vi "VI AK TCP.vi"(5 "Port changed in":bool, 6 "Aktionen":T1, 8 "error in":errorcluster caption="error out", 10 "Port":u16=3615, 11 "Sprachliste":string[][](array[string])) -> (0 "error out":errorcluster, 3 "connection ID":refnum<k5>)   [LabVIEW 2020, in "AK-Schnittstelle.lvlib" / "AK TCP.lvlib"]
uses:
  AK TCP.lvlib
  Aktionen AK.ctl
  Daten weitergeben Aktionen.ctl
  Aktionen Gespeicherte Werte.ctl
  AK-Schnittstelle.lvlib
  Sprachverwaltung/Sprachverwaltung.lvlib
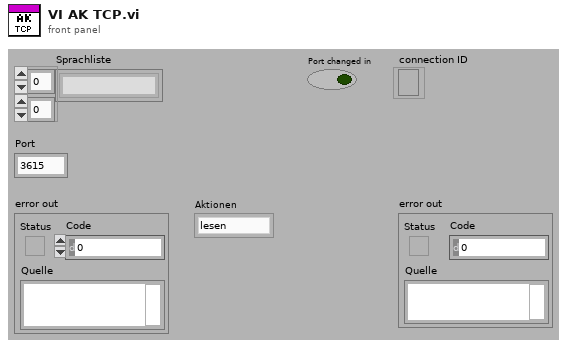
[diagram p1: front panel]
types:
  T1 = typedef "AK-Schnittstelle.lvlib/Aktionen AK.ctl" = enum16{"lesen", "initialisieren", "beenden", "AK Komm"}
  T2 = typedef "AK-Schnittstelle.lvlib/Daten weitergeben Aktionen.ctl" = enum16{"lesen", "schreiben", "Log löschen", "Detail", "Detail löschen", "Speicher Freigeben"}
  T3 = typedef "AK-Schnittstelle.lvlib/Aktionen Gespeicherte Werte.ctl" = enum16{"lesen", "laden", "speichern", "Seriell", "TCP", "Diverse", "AKTIV", "AK-Namen"}
  T4 = typedef "AK-Schnittstelle.lvlib/Diverse gespeicherte Werte.ctl" = cluster{"Kalibriergaseingang":i16, "SamplePoint":i16, "CalGas zu PNS":i16, "Gas-Reihenfolge":i16[], "Zeit 0-Gas":sgl, "Zeit CalGas":sgl, "AK Befehlssatz":T5}
  T5 = typedef "AK-Schnittstelle.lvlib/AK Befehlssatz.ctl" = enum16{"MEXA", "IAG v1.4", "AVL (Puma)", "PEUS"}
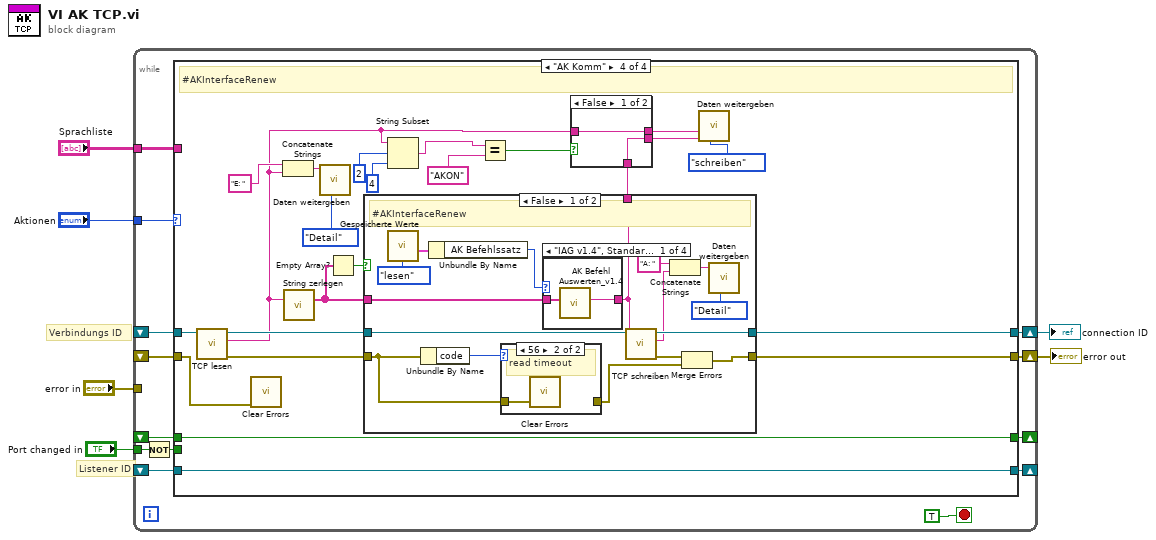
[diagram p0: block diagram]
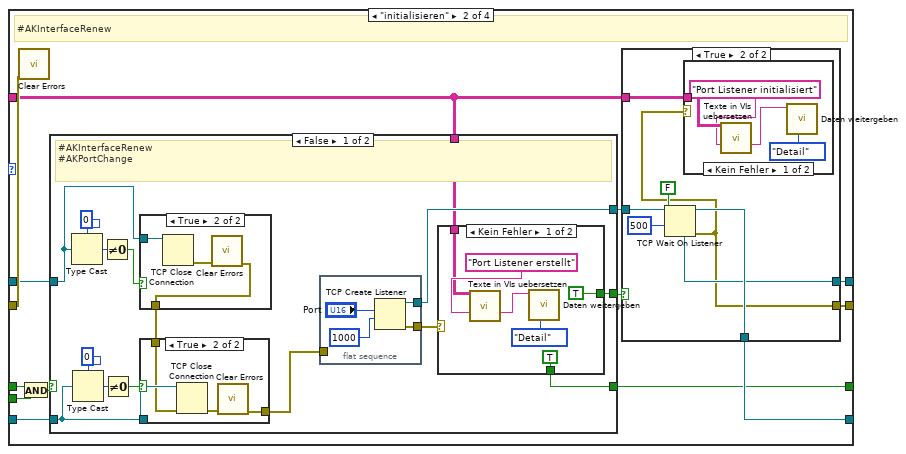
[diagram p3: hidden frame]
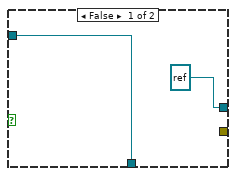
[diagram p4: hidden frame]
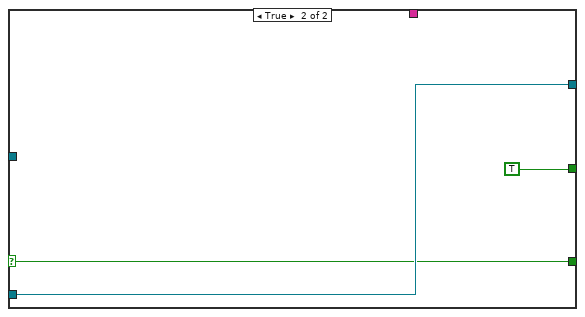
[diagram p9: hidden frame]
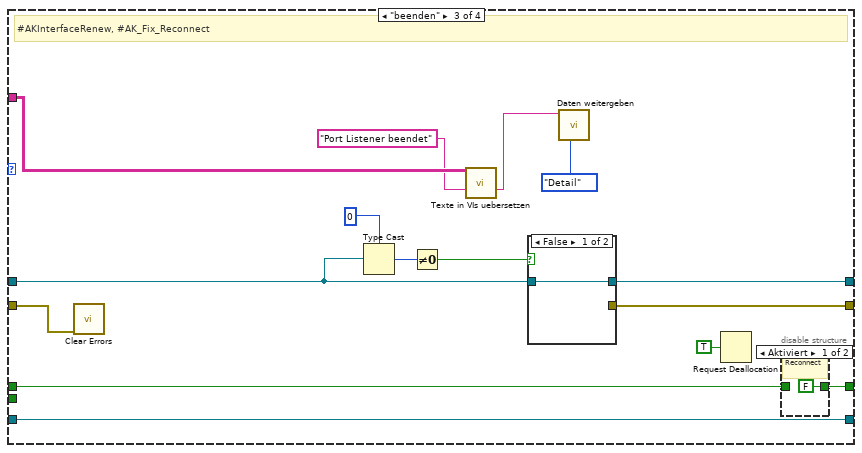
[diagram p10: hidden frame]
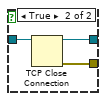
[diagram p11: hidden frame]
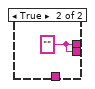
[diagram p13: hidden frame]
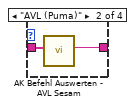
[diagram p15: hidden frame]
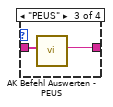
[diagram p16: hidden frame]
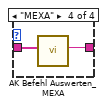
[diagram p17: hidden frame]
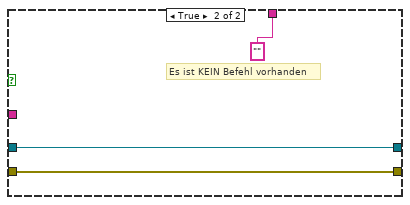
[diagram p18: hidden frame]
diagram:
  # "Verbindungs ID"
  # "Listener ID"
  n1 = while {
    tunnel: "Aktionen" -> [w19]
    shift-right: [w17] -> _
    shift-left: _ -> [w16]
    shift-right: [w18] -> w5
    shift-left: _ -> [w15]
    tunnel: "error in" -> [_]
    shift-right: [w13] -> w3
    shift-left: _ -> [w12]
    shift-right: [w10] -> _
    shift-left: _ -> [w11]
    tunnel: "Port changed in" -> [w9]
    tunnel: "Sprachliste" -> [w7]
    stop <- TRUE stop-if-true
    n2 = Not(x=w9) -> (.not. x?=w8:bool)
    n3 = case shown="\"AK Komm\"" w19 {
      tunnel: [w22 w30 w99 w126] -> w18
      tunnel: [w23 w35 w97 w120] -> w17
      tunnel: w16 -> [w23 w34 w97 w120]
      tunnel: w15 -> [w22 w31 w96 w123]
      tunnel: [w21 w33 w98 w119] -> w13
      tunnel: w12 -> [w21 w26 w89 w121]
      tunnel: w11 -> [w20 w29 w92 w118]
      tunnel: [w20 w32 w93 w118] -> w10
      tunnel: w8 -> [_ w28 _ _]
      tunnel: w7 -> [_ w24 w87 _]
      frame "lesen", Default {
      }
      frame "initialisieren" {
        # "#AKInterfaceRenew"
        n4 = call <vilib>:"Clear Errors.vi"("error in (no error)"=w31) -> ()  [unwired: 5 in, 2 out]
        n5 = And(x=w29, y=w28) -> (x .and. y?=w27:bool)
        n6 = case shown="False" w27 {
          selector: w27 -> [_ w83]
          tunnel: [w64 w84] -> w36
          tunnel: w34 -> [w60 w84]
          tunnel: [w62 w83] -> w32
          tunnel: w26 -> [w54 _]
          tunnel: [w51 TRUE] -> w25
          tunnel: w24 -> [w50 _]
          frame False {
            # "#AKInterfaceRenew\n#AKPortChange"
            n7 = Type Cast(type=u32 0, x=w54) -> (*(type *) &x=w57:u32)
            n8 = Type Cast(type=u32 0, x=w60) -> (*(type *) &x=w61:u32)
            n9 = Not Equal To 0?(x=w57) -> (x != 0?=w55:bool)
            n10 = Not Equal To 0?(x=w61) -> (x != 0?=w59:bool)
            n11 = case shown="True" w55 {
              tunnel: [_ w66] -> w53
              tunnel: w54 -> [_ w65]
              frame False {
              }
              frame True {
                n12 = TCP Close Connection(connection ID=w65) -> (error out=w67:errorcluster)  [unwired: 2 in, 1 out]
                n13 = call <vilib>:"Clear Errors.vi"("error in (no error)"=w67) -> ("error out"=w66:errorcluster)  [unwired: 5 in, 1 out]
              }
            }
            n14 = case shown="True" w59 {
              tunnel: w60 -> [_ w71]
              tunnel: w53 -> [_ w69]
              tunnel: [_ w68] -> w52
              frame False {
              }
              frame True {
                n15 = TCP Close Connection(connection ID=w71, error in (no error)=w69) -> (error out=w70:errorcluster)  [unwired: 1 in, 1 out]
                n16 = call <vilib>:"Clear Errors.vi"("error in (no error)"=w70) -> ("error out"=w68:errorcluster)  [unwired: 5 in, 1 out]
              }
            }
            n17 = flat-sequence {
              tunnel: [w74] -> w64
              tunnel: [w73] -> w63
              tunnel: w52 -> [_]
              frame #0 {
                n18 = TCP Create Listener(9:1000 ("timeout ms (wait forever: -1)"), 10:"Port") -> (0:w73:errorcluster, 3:w74:refnum<k5>)  [unwired: 3 in, 1 out]
              }
            }
            n19 = case shown="Kein Fehler" w63 {
              tunnel: [TRUE _] -> w62
              tunnel: [TRUE _] -> w51
              tunnel: w50 -> [w77 _]
              frame No Error {
                n20 = call "Texte in VIs uebersetzen.vi"("Sprachliste"=w77, "String zum Übersetzen"="Port Listener erstellt" ("Detail")) -> ("String zum Übersetzen"=w76:string)  [unwired: 9 in, 4 out]
                n21 = call "Daten weitergeben.vi"("Aktionen"=Daten_weitergeben_Aktionen."Detail", "Detail"=w76) -> ()  [unwired: 5 in, 5 out]
              }
              frame Error {
              }
            }
          }
          frame True {
          }
        }
        n22 = case shown="True" w25 {
          tunnel: w36 -> [w38 w44]
          tunnel: [w38 w43] -> w35
          tunnel: [refnum<k5> refnum ("listener ID") w42] -> w33
          tunnel: [_ w40] -> w30
          tunnel: w24 -> [_ w39]
          frame False {
          }
          frame True {
            n23 = TCP Wait On Listener(9:500 ("Timeout in ms (kein: -1)"), 10:FALSE ("Auflösen der Netzwerkadresse (T)"), 11:w44) -> (0:w40:errorcluster, 3:w43:refnum<k5>, 4:w42:refnum<k5>)  [unwired: 1 in, 2 out]
            n24 = case shown="Kein Fehler" w40 {
              tunnel: w39 -> [w48 _]
              frame No Error {
                n25 = call "Texte in VIs uebersetzen.vi"("Sprachliste"=w48, "String zum Übersetzen"="Port Listener initialisiert" ("Detail")) -> ("String zum Übersetzen"=w46:string)  [unwired: 9 in, 4 out]
                n26 = call "Daten weitergeben.vi"("Aktionen"=Daten_weitergeben_Aktionen."Detail", "Detail"=w46) -> ()  [unwired: 5 in, 5 out]
              }
              frame Error {
              }
            }
          }
        }
      }
      frame "beenden" {
        # "#AKInterfaceRenew, #AK_Fix_Reconnect"
        n27 = call <vilib>:"Clear Errors.vi"("error in (no error)"=w96) -> ()  [unwired: 5 in, 2 out]
        n28 = Type Cast(type=u32 0, x=w89) -> (*(type *) &x=w91:u32)
        n29 = Not Equal To 0?(x=w91) -> (x != 0?=w88:bool)
        n30 = call "Texte in VIs uebersetzen.vi"("Sprachliste"=w87, "String zum Übersetzen"="Port Listener beendet" ("Detail")) -> ("String zum Übersetzen"=w85:string)  [unwired: 9 in, 4 out]
        n31 = case shown="False" w88 {
          tunnel: [_ w103] -> w99
          tunnel: w89 -> [w100 w102]
          tunnel: [w100 w101] -> w98
          frame False {
          }
          frame True {
            n32 = TCP Close Connection(connection ID=w102) -> (connection ID out=w101:refnum<k5>, error out=w103:errorcluster)  [unwired: 2 in]
          }
        }
        n33 = call "Daten weitergeben.vi"("Aktionen"=Daten_weitergeben_Aktionen."Detail", "Detail"=w85) -> ()  [unwired: 5 in, 5 out]
        n34 = Request Deallocation(TRUE ("Flag")) -> ()
        n35 = disable-structure shown="Aktiviert" {
          disable-tunnel: [FALSE w105] -> w93
          disable-tunnel: w92 -> [_ w105]
          frame Enabled {
            # "#AK_Fix_Reconnect"
          }
          frame Disabled {
          }
        }
      }
      frame "AK Komm" {
        # "#AKInterfaceRenew"
        n36 = call "TCP lesen.vi"("connection ID"=w121) -> ("error out"=w122:errorcluster, "Daten (Ausgang)"=w109:string, "connection ID"=w125:refnum<k5>)  [unwired: 8 in]
        n37 = call <vilib>:"Clear Errors.vi"("error in (no error)"=w123) -> ()  [unwired: 5 in, 2 out]
        n38 = Concatenate Strings("E: ", w109) -> (w116:string)
        n39 = call "String zerlegen.vi"("read buffer"=w109) -> ("Array"=w128:string[])  [unwired: 14 in]
        n40 = call "Daten weitergeben.vi"("Aktionen"=Daten_weitergeben_Aktionen."Detail", "Detail"=w116) -> ()  [unwired: 5 in, 5 out]
        n41 = Empty Array?(array=w128) -> (empty?=w127:bool)
        n42 = case shown="False" w127 {
          tunnel: w128 -> [w145 _]
          tunnel: w125 -> [w147 w160]
          tunnel: [w146 w160] -> w119
          tunnel: [w135 w158] -> w126
          tunnel: w122 -> [w133 w158]
          tunnel: [w144 "" ("String für schreiben")] -> w111
          frame False {
            # "#AKInterfaceRenew"
            n43 = call "Gespeicherte Werte.vi"("Aktionen"=Aktionen_Gespeicherte_Werte."lesen") -> ("Diverse Werte"=w142:T4)  [unwired: 6 in, 4 out]
            n44 = Unbundle By Name(w133) -> ("code"=w132:i32)
            n45 = Unbundle By Name(w142) -> ("AK Befehlssatz"=w141:T5)
            n46 = case shown="56" w132 {
              tunnel: w133 -> [w148 w149]
              tunnel: [w148 _] -> w134
              frame Default {
              }
              frame 56 {
                # "read timeout"
                n47 = call <vilib>:"Clear Errors.vi"("error in (no error)"=w149) -> ()  [unwired: 5 in, 2 out]
              }
            }
            n48 = case shown="\"IAG v1.4\", Standard" w141 {
              tunnel: w145 -> [w151 w153 w154 w157]
              tunnel: [w150 w152 w155 w156] -> w144
              frame "IAG v1.4", Default {
                n49 = call "AK Befehl Auswerten_v1.4.vi"("Array"=w151) -> ("String für schreiben"=w150:string)  [unwired: 10 in]
              }
              frame "AVL (Puma)" {
                n50 = call "AK Befehl Auswerten - AVL Sesam.vi"("Array"=w153) -> ("String für schreiben"=w152:string)  [unwired: 10 in]
              }
              frame "PEUS" {
                n51 = call "AK Befehl Auswerten - PEUS.vi"("Array"=w154) -> ("String für schreiben"=w155:string)  [unwired: 10 in]
              }
              frame "MEXA" {
                n52 = call "AK Befehl Auswerten_MEXA.vi"("Array"=w157) -> ("String für schreiben"=w156:string)  [unwired: 10 in]
              }
            }
            n53 = call "TCP schreiben.vi"("String"=w144, "connection ID"=w147) -> ("error out"=w136:errorcluster, "Verknüpfter String"=w137:string, "connection ID"=w146:refnum<k5>)  [unwired: 7 in]
            n54 = Concatenate Strings("A: " ("String"), w137) -> (w139:string)
            n55 = Merge Errors(w136, w134) -> (w135:errorcluster)
            n56 = call "Daten weitergeben.vi"("Aktionen"=Daten_weitergeben_Aktionen."Detail", "Detail"=w139) -> ()  [unwired: 5 in, 5 out]
          }
          frame True {
            # "Es ist KEIN Befehl vorhanden"
          }
        }
        n57 = String Subset(string=w109, offset (0)=2 ("Offset (0)"), length (rest)=4 ("Länge (Rest)")) -> (substring=w107:string)
        n58 = Equal?(x=w107, y="AKON") -> (x = y?=w113:bool)
        n59 = case shown="False" w113 {
          tunnel: w109 -> [w130 _]
          tunnel: [w130 w131] -> w112
          tunnel: w111 -> [w129 _]
          tunnel: [w129 w131] -> w110
          frame False {
          }
          frame True {
            w131 = "" ("Daten (Ausgang)")
          }
        }
        n60 = call "Daten weitergeben.vi"("Aktionen"=Daten_weitergeben_Aktionen."schreiben", "Antwort"=w110, "Empfangspuffer"=w112) -> ()  [unwired: 4 in, 5 out]
      }
    }
  }
  "error out" <- w5
  "connection ID" <- w3
